vi "move.vi"(8 "delay":u32, 9 "Enum":T1(ring), 10 "D":dbl) -> ()   [LabVIEW 2017]
uses:
  Constant.vi
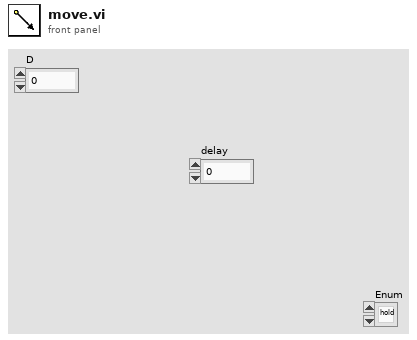
[diagram p1: front panel]
types:
  T1 = enum16{"hold", "f", "fl", "fr", "l", "r", "b", "bl", "br"}
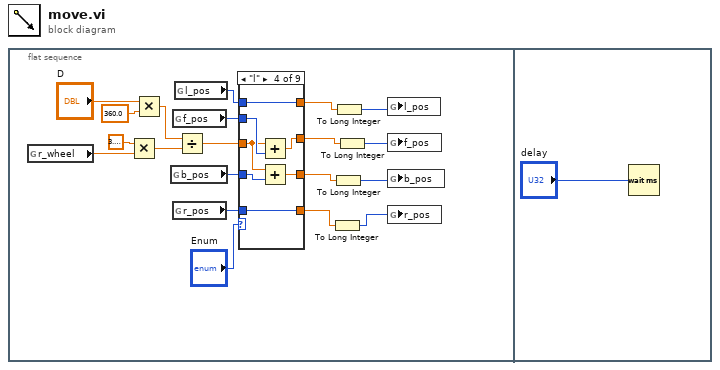
[diagram p0: block diagram]
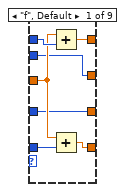
[diagram p2: hidden frame]
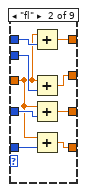
[diagram p3: hidden frame]
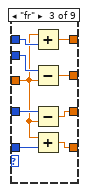
[diagram p4: hidden frame]
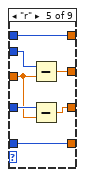
[diagram p5: hidden frame]
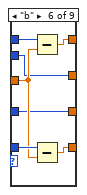
[diagram p6: hidden frame]
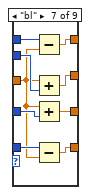
[diagram p7: hidden frame]
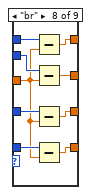
[diagram p8: hidden frame]
diagram:
  n1 = flat-sequence {
    frame #0 {
      n2 = global read "Constant.vi" "r_wheel"() -> (w20:dbl)
      n3 = Multiply(x=3.141592653589793, y=w20) -> (x*y=w15:dbl)
      n4 = Multiply(x="D", y=360.0) -> (x*y=w16:dbl)
      n5 = global read "Constant.vi" "b_pos"() -> (w9:i32)
      n6 = global read "Constant.vi" "f_pos"() -> (w10:i32)
      n7 = global read "Constant.vi" "r_pos"() -> (w11:i32)
      n8 = global read "Constant.vi" "l_pos"() -> (w12:i32)
      n9 = Divide(x=w16, y=w15) -> (x/y=w13:dbl)
      n10 = case shown="\"l\"" "Enum" {
        tunnel: [w24 w31 w43 w47 w54 w66 w73 w84 w88] -> w7
        tunnel: w13 -> [w25 w32 w37 w50 w55 w62 w67 w76 _]
        tunnel: [w23 w30 w42 w46 w53 w65 w72 w83 w85] -> w2
        tunnel: [w22 w29 w41 w49 w59 w61 w71 w82 w87] -> w6
        tunnel: [w21 w28 w40 w48 w58 w60 w70 w81 w86] -> w4
        tunnel: w12 -> [w27 w33 w45 w47 w54 w64 w68 w80 w88]
        tunnel: w11 -> [w26 w34 w44 w46 w53 w63 w69 w77 w85]
        tunnel: w10 -> [w22 w36 w39 w52 w57 w61 w75 w79 w87]
        tunnel: w9 -> [w21 w35 w38 w51 w56 w60 w74 w78 w86]
        frame "f", Default {
          n11 = Add(x=w25, y=w27) -> (x+y=w24:dbl)
          n12 = Add(x=w25, y=w26) -> (x+y=w23:dbl)
        }
        frame "fl" {
          n13 = Add(x=w32, y=w33) -> (x+y=w31:dbl)
          n14 = Add(x=w32, y=w36) -> (x+y=w29:dbl)
          n15 = Add(x=w32, y=w35) -> (x+y=w28:dbl)
          n16 = Add(x=w32, y=w34) -> (x+y=w30:dbl)
        }
        frame "fr" {
          n17 = Add(x=w37, y=w45) -> (x+y=w43:dbl)
          n18 = Subtract(x=w39, y=w37) -> (x-y=w41:dbl)
          n19 = Subtract(x=w38, y=w37) -> (x-y=w40:dbl)
          n20 = Add(x=w37, y=w44) -> (x+y=w42:dbl)
        }
        frame "l" {
          n21 = Add(x=w50, y=w52) -> (x+y=w49:dbl)
          n22 = Add(x=w50, y=w51) -> (x+y=w48:dbl)
        }
        frame "r" {
          n23 = Subtract(x=w57, y=w55) -> (x-y=w59:dbl)
          n24 = Subtract(x=w56, y=w55) -> (x-y=w58:dbl)
        }
        frame "b" {
          n25 = Subtract(x=w64, y=w62) -> (x-y=w66:dbl)
          n26 = Subtract(x=w63, y=w62) -> (x-y=w65:dbl)
        }
        frame "bl" {
          n27 = Subtract(x=w68, y=w67) -> (x-y=w73:dbl)
          n28 = Add(x=w67, y=w75) -> (x+y=w71:dbl)
          n29 = Add(x=w67, y=w74) -> (x+y=w70:dbl)
          n30 = Subtract(x=w69, y=w67) -> (x-y=w72:dbl)
        }
        frame "br" {
          n31 = Subtract(x=w80, y=w76) -> (x-y=w84:dbl)
          n32 = Subtract(x=w79, y=w76) -> (x-y=w82:dbl)
          n33 = Subtract(x=w78, y=w76) -> (x-y=w81:dbl)
          n34 = Subtract(x=w77, y=w76) -> (x-y=w83:dbl)
        }
        frame "hold" {
        }
      }
      n35 = To Long Integer(number=w2) -> (32bit integer=w1:i32)
      n36 = To Long Integer(number=w4) -> (32bit integer=w3:i32)
      n37 = To Long Integer(number=w7) -> (32bit integer=w8:i32)
      n38 = To Long Integer(number=w6) -> (32bit integer=w5:i32)
      n39 = global write "Constant.vi" "l_pos"(w8) -> ()
      n40 = global write "Constant.vi" "f_pos"(w5) -> ()
      n41 = global write "Constant.vi" "b_pos"(w3) -> ()
      n42 = global write "Constant.vi" "r_pos"(w1) -> ()
    }
    frame #1 {
      n43 = Wait (ms)(milliseconds to wait="delay") -> ()  [unwired: 1 out]
    }
  }
